vi "Module Name--constant.vi"() -> (3 "Module Name":string)   [LabVIEW 2020, in "TCP_Server.lvlib"]
doc: "Return the name of the module that owns this VI. \n_____\nBased on DQMH Project Template 6.0.0.91."
uses:
  TCP_Server.lvlib
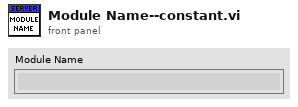
[diagram p1: front panel]
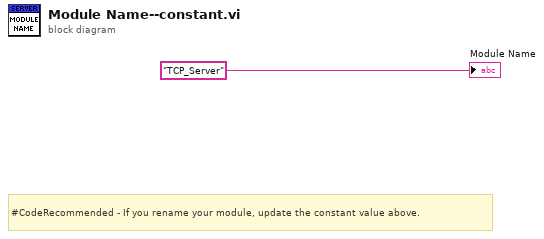
[diagram p0: block diagram]
diagram:
  # "#CodeRecommended - If you rename your module, update the constant value above."
  "Module Name" <- "TCP_Server"
